vi "Delete Topic.vi"(8 "error in (no error)":errorcluster, 11 "Topic":refnum<class "Topic.lvclass">) -> (0 "error out":errorcluster)   [LabVIEW 2015, in "NI_AWS_SNS.lvlib" / "Topic.lvclass"]
uses:
  Topic.lvclass
  Core/ARN/ARN.lvclass
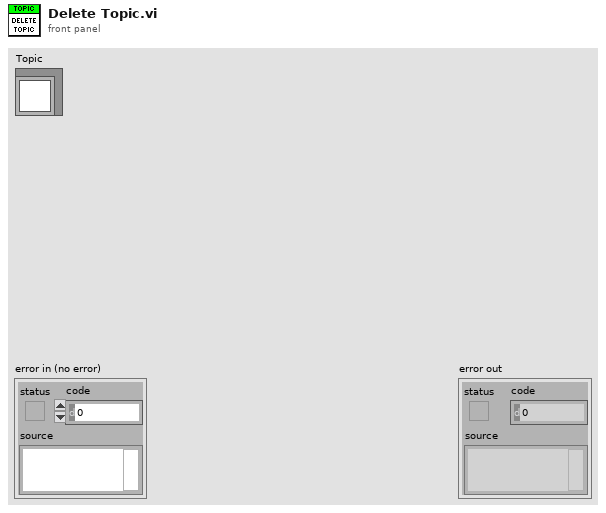
[diagram p1: front panel]
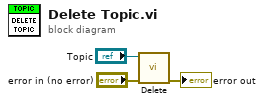
[diagram p0: block diagram]
diagram:
  n1 = call "Delete.vi"("error in (no error)"="error in (no error)", "ARN in"="Topic") -> ("error out"=→"error out":errorcluster)  [unwired: 9 in]
